vi "4 PulseGenerations.vi"(2 "PulseGen Packets":u64[](array[numeric])=[0, 0, 0, 0], 4 "4 PulseGen Chs":T1={"DO0"="NI 9474/DO0", "DO1"="NI 9474/DO1", "DO2"="NI 9474/DO2", "DO3"="NI 9474/DO3"}) -> ()   [LabVIEW 2010]
uses:
  <vilib>/eio/EIONode/EIONode.xnode
  <vilib>/rvi/eio/nirviEIOImplementation/nirviEIOImplementation.xnode
  <vilib>/rvi/eio/common/nirviEmuClasses.ctl
  <vilib>/rvi/eio/common/nirviEmuTemplateMethod_noerrors.vi
  <vilib>/NI Veristand/FPGA/NI_VS FPGA Support.lvlib
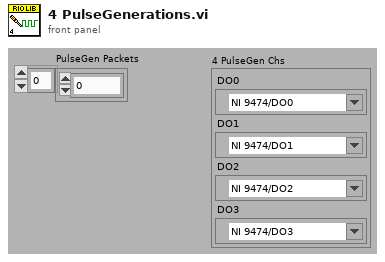
[diagram p1: front panel]
types:
  T1 = cluster{"DO0":refnum<k21>, "DO1":refnum<k21>, "DO2":refnum<k21>, "DO3":refnum<k21>}
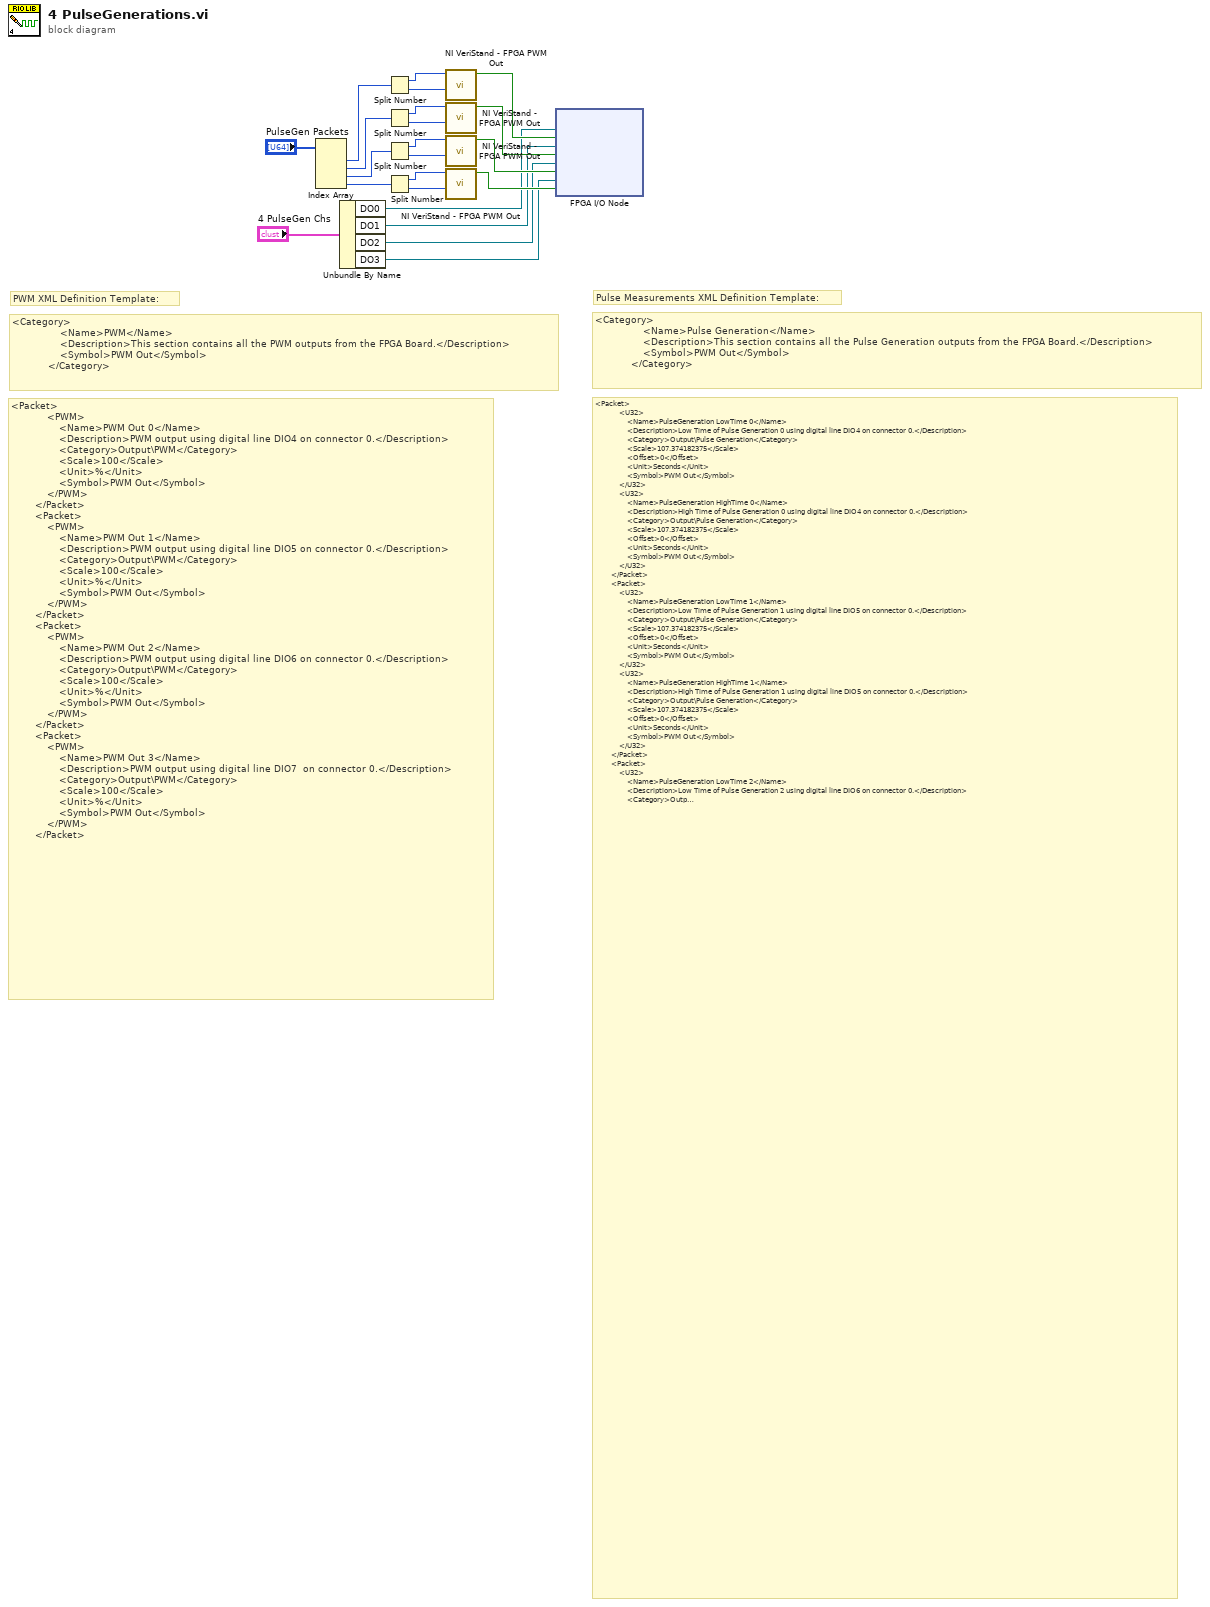
[diagram p0: block diagram]
diagram:
  # "<Category>\n                <Name>Pulse Generation</Name>\n                <Description>This section contains all the Pulse Generation outputs from the FPGA Board.</Description>\n                <Symbol>PWM Out</Symbol>\n            </Category>"
  # "<Category>\n                <Name>PWM</Name>\n                <Description>This section contains all the PWM outputs from the FPGA Board.</Description>\n                <Symbol>PWM Out</Symbol>\n            </Category>"
  # "<Packet>\n            <U32>\n                <Name>PulseGeneration LowTime 0</Name>\n                <Description>Low Time of Pulse Generation 0 using digital line DIO4 on connector 0.</Description>\n                <Category>Output\\Pulse Generation</Category>\n                <Scale>107.374182375</Scale>\n                <Offset>0</Offset>\n                <Unit>Seconds</Unit>\n                <Symbol>PWM Out</Symbol>\n            </U32>\n            <U32>\n                <Name>PulseGeneration HighTime 0</Name>\n                <Description>High Time of Pulse Generation 0 using digital line DIO4 on connector 0.</Description>\n                <Category>Output\\Pulse Generation</Category>\n                <Scale>107.374182375</Scale>\n                <Offset>0</Offset>\n                <Unit>Seconds</Unit>\n                <Symbol>PWM Out</Symbol>\n            </U32>\n        </Packet>\n        <Packet>\n            <U32>\n                <Name>PulseGeneration LowTime 1</Name>\n                <Description>Low Time of Pulse Generation 1 using digital line DIO5 on connector 0.</Description>\n                <Category>Output\\Pulse Generation</Category>\n                <Scale>107.374182375</Scale>\n                <Offset>0</Offset>\n                <Unit>Seconds</Unit>\n                <Symbol>PWM Out</Symbol>\n            </U32>\n            <U32>\n                <Name>PulseGeneration HighTime 1</Name>\n                <Description>High Time of Pulse Generation 1 using digital line DIO5 on connector 0.</Description>\n                <Category>Output\\Pulse Generation</Category>\n                <Scale>107.374182375</Scale>\n                <Offset>0</Offset>\n                <Unit>Seconds</Unit>\n                <Symbol>PWM Out</Symbol>\n            </U32>\n        </Packet>\n        <Packet>\n            <U32>\n                <Name>PulseGeneration LowTime 2</Name>\n                <Description>Low Time of Pulse Generation 2 using digital line DIO6 on connector 0.</Description>\n                <Category>Output\\Pulse Generation</Category>\n                <Scale>107.374182375</Scale>\n                <Offset>0</Offset>\n                <Unit>Seconds</Unit>\n                <Symbol>PWM Out</Symbol>\n            </U32>\n            <U32>\n                <Name>PulseGeneration HighTime 2</Name>\n                <Description>High Time of Pulse Generation 2 using digital line DIO6 on connector 0.</Description>\n                <Category>Output\\Pulse Generation</Category>\n                <Scale>107.374182375</Scale>\n                <Offset>0</Offset>\n                <Unit>Seconds</Unit>\n                <Symbol>PWM Out</Symbol>\n            </U32>\n        </Packet>\n        <Packet>\n            <U32>\n                <Name>PulseGeneration LowTime 3</Name>\n                <Description>Low Time of Pulse Generation 3 using digital line DIO7 on connector 0.</Description>\n                <Category>Output\\Pulse Generation</Category>\n                <Scale>107.374182375</Scale>\n                <Offset>0</Offset>\n                <Unit>Seconds</Unit>\n                <Symbol>PWM Out</Symbol>\n            </U32>\n            <U32>\n                <Name>PulseGeneration HighTime 3</Name>\n                <Description>High Time of Pulse Generation 3 using digital line DIO7 on connector 0.</Description>\n                <Category>Output\\Pulse Generation</Category>\n                <Scale>107.374182375</Scale>\n                <Offset>0</Offset>\n                <Unit>Seconds</Unit>\n                <Symbol>PWM Out</Symbol>\n            </U32>\n        </Packet>"
  # "Pulse Measurements XML Definition Template:"
  # "<Packet>\n            <PWM>\n                <Name>PWM Out 0</Name>\n                <Description>PWM output using digital line DIO4 on connector 0.</Description>\n                <Category>Output\\PWM</Category>\n                <Scale>100</Scale>\n                <Unit>%</Unit>\n                <Symbol>PWM Out</Symbol>\n            </PWM>\n        </Packet>\n        <Packet>\n            <PWM>\n                <Name>PWM Out 1</Name>\n                <Description>PWM output using digital line DIO5 on connector 0.</Description>\n                <Category>Output\\PWM</Category>\n                <Scale>100</Scale>\n                <Unit>%</Unit>\n                <Symbol>PWM Out</Symbol>\n            </PWM>\n        </Packet>\n        <Packet>\n            <PWM>\n                <Name>PWM Out 2</Name>\n                <Description>PWM output using digital line DIO6 on connector 0.</Description>\n                <Category>Output\\PWM</Category>\n                <Scale>100</Scale>\n                <Unit>%</Unit>\n                <Symbol>PWM Out</Symbol>\n            </PWM>\n        </Packet>\n        <Packet>\n            <PWM>\n                <Name>PWM Out 3</Name>\n                <Description>PWM output using digital line DIO7  on connector 0.</Description>\n                <Category>Output\\PWM</Category>\n                <Scale>100</Scale>\n                <Unit>%</Unit>\n                <Symbol>PWM Out</Symbol>\n            </PWM>\n        </Packet>"
  # "PWM XML Definition Template:"
  n1 = Index Array(array="PulseGen Packets") -> (element #1=w17:u64, element #2=w18:u64, element #3=w19:u64, element #4=w20:u64)  [unwired: 4 in]
  n2 = Unbundle By Name("4 PulseGen Chs") -> ("DO0"=w1:refnum<k21>, "DO1"=w4:refnum<k21>, "DO2"=w3:refnum<k21>, "DO3"=w2:refnum<k21>)
  n3 = Split Number(x=w17) -> (hi(x)=w7:u32, lo(x)=w8:u32)
  n4 = Split Number(x=w18) -> (hi(x)=w10:u32, lo(x)=w9:u32)
  n5 = Split Number(x=w19) -> (hi(x)=w11:u32, lo(x)=w12:u32)
  n6 = Split Number(x=w20) -> (hi(x)=w14:u32, lo(x)=w13:u32)
  n7 = call <vilib>:"NI VeriStand - FPGA PWM Out.vi"("_Low Time"=w8, "_High Time"=w7) -> ("Output"=w6:bool)  [unwired: 1 in, 8 out]
  n8 = call <vilib>:"NI VeriStand - FPGA PWM Out.vi"("_Low Time"=w9, "_High Time"=w10) -> ("Output"=w21:bool)  [unwired: 1 in, 8 out]
  n9 = call <vilib>:"NI VeriStand - FPGA PWM Out.vi"("_Low Time"=w12, "_High Time"=w11) -> ("Output"=w22:bool)  [unwired: 1 in, 8 out]
  n10 = call <vilib>:"NI VeriStand - FPGA PWM Out.vi"("_Low Time"=w13, "_High Time"=w14) -> ("Output"=w15:bool)  [unwired: 1 in, 8 out]
  n11 = xnode "FPGA I/O Node"("I/O Item"=w6, "I/O Item"=w21, "I/O Item"=w22, "I/O Item"=w15, "FPGA I/O In"=w1, "FPGA I/O In"=w4, "FPGA I/O In"=w3, "FPGA I/O In"=w2) -> ()  [unwired: 4 out]
